vi "Shortcuts.vi"() -> (3 "DAQmx Shortcuts":T1[](array[typedef])=[{"DAQmx Global Channel"="Mixer_Channel1_Level", "Message Queue"="Mixer", "Event"="Value Change", "Target"="Crossfader", "Momentary"=FALSE, "Data"=variant}, {"DAQmx Global Channel"="Deck1_Play", "Message Queue"="Deck1", "Event"="Value Change", "Target"="Play", "Momentary"=FALSE, "Data"=variant}])   [LabVIEW 2018, in "DAQmx.lvlib"]
uses:
  DAQmx.lvlib
  DAQmx Shortcut.ctl
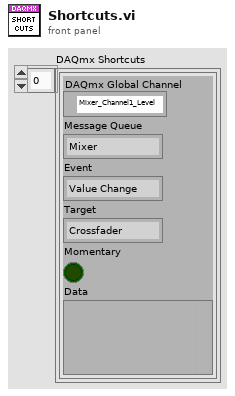
[diagram p1: front panel]
types:
  T1 = typedef "DAQmx.lvlib/DAQmx Shortcut.ctl" = cluster{"DAQmx Global Channel":refnum<k21>, "Message Queue":string, "Event":string, "Target":string, "Momentary":bool, "Data":variant}
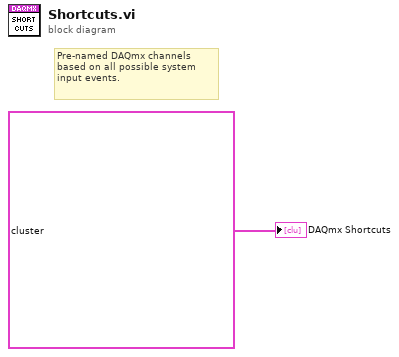
[diagram p0: block diagram]
diagram:
  # "Pre-named DAQmx channels based on all possible system input events."
  "DAQmx Shortcuts" <- T1[] [{"DAQmx Global Channel"="Mixer_Channel1_Level", "Message Queue"="Mixer", "Event"="Value Change", "Target"="Crossfader", "Momentary"=FALSE, "Data"=variant}, {"DAQmx Global Channel"="Deck1_Play", "Message Queue"="Deck1", "Event"="Value Change", "Target"="Play", "Momentary"=FALSE, "Data"=variant}]
